vi "3.vi"() -> ()   [LabVIEW 2017]
panel:
  in  "旋钮":dbl(knob) scale=0.2..1.0
  in  "停止":bool
  out "布尔 2":bool
  out "布尔":bool
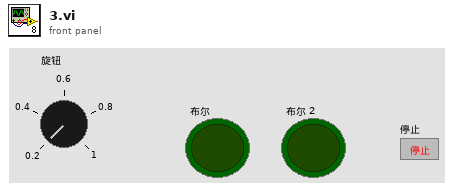
[diagram p1: front panel]
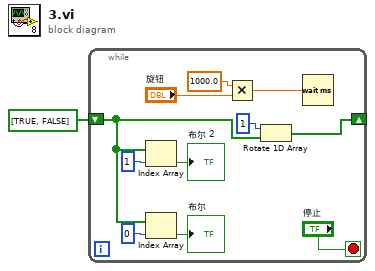
[diagram p0: block diagram]
diagram:
  n1 = while {
    shift-right: [w10] -> _
    shift-left: bool[] [TRUE, FALSE] -> [w6]
    stop <- "停止" stop-if-true
    n2 = Index Array(array=w6, index=1 ("索引")) -> (element=→"布尔 2":bool)
    n3 = Index Array(array=w6, index=0 ("索引")) -> (element=→"布尔":bool)
    n4 = Multiply(x=1000.0, y="旋钮") -> (x*y=w2:dbl)
    n5 = Rotate 1D Array(1:w6, 2:1 ("n")) -> (0:w10:bool[])
    n6 = Wait (ms)(milliseconds to wait=w2) -> ()  [unwired: 1 out]
  }
